vi "Canny Edge.vi"(4 "Threshold 2":dbl=100.0, 6 "Threshold 1":dbl=50.0, 7 "Aperture Size":T1, 8 "error in (no error)":errorcluster, 10 "Canny Edge Result":T2, 11 "Greyscale Image-Source":T2) -> (0 "error out":errorcluster, 3 "Canny Edge (duplicate)":T2)   [LabVIEW 2020, in "image.lvlib"]
uses:
  image.lvlib
  Greyscale Image.ctl
  Canny Aperture Size.ctl
  common/common.lvlib
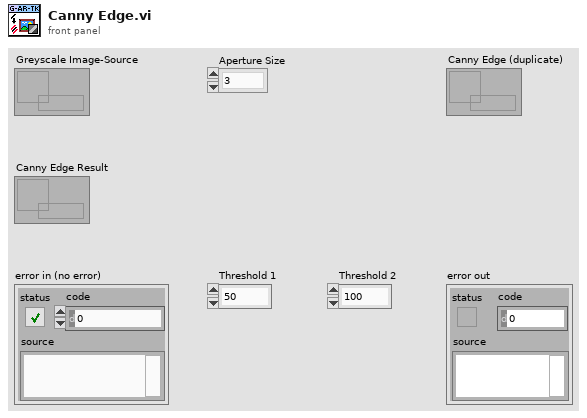
[diagram p1: front panel]
types:
  T1 = typedef "image.lvlib/Canny Aperture Size.ctl" = enum16{"3", "5", "7"}
  T2 = typedef "image.lvlib/Greyscale Image.ctl" = refnum<data-value>
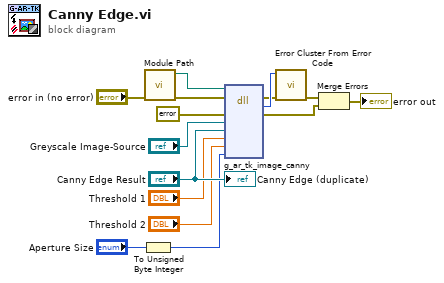
[diagram p0: block diagram]
diagram:
  n1 = To Unsigned Byte Integer(number="Aperture Size") -> (unsigned 8bit integer=w5:u8)
  n2 = call "Module Path.vi"("error in (no error)"="error in (no error)") -> ("error out"=w2:errorcluster, "Path"=w1:path)  [unwired: 9 in]
  n3 = dll-call lib="?" fn="g_ar_tk_image_canny" ("g_ar_toolkit.*.*:g_ar_tk_image_in_range")(path in=w1, error in=w2, "error_cluster"=errorcluster {"status"=FALSE, "code"=0, "source"=""} ("error constant"), "EDVR src"="Greyscale Image-Source", "EDVR dst"="Canny Edge Result", "threshold_1"="Threshold 1", "threshold_2"="Threshold 2", "aperture_size"=w5) -> (error out=w6:errorcluster, "MgErr"=w7:i32, "error_cluster"=w10:errorcluster)  [unwired: 6 in, 1 out]
  n4 = call <vilib>:"Error Cluster From Error Code.vi"("error in (no error)"=w6, "error code (0)"=w7) -> ("error out"=w8:errorcluster)  [unwired: 7 in]
  n5 = Merge Errors(w8, w10) -> (→"error out":errorcluster)
  "Canny Edge (duplicate)" <- "Canny Edge Result"
